vi "Parse Target ID.vi"(11 "targetID":string) -> (0 "target location":string, 3 "target name":string)   [LabVIEW 2020, in "NI_TargetHelper.lvlib"]
uses:
  <vilib>/TargetSupport/NI_TargetHelper/NI_TargetHelper.lvlib
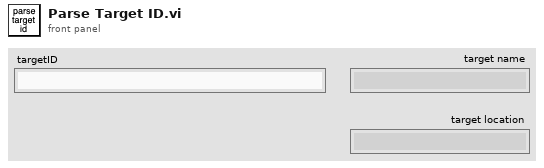
[diagram p1: front panel]
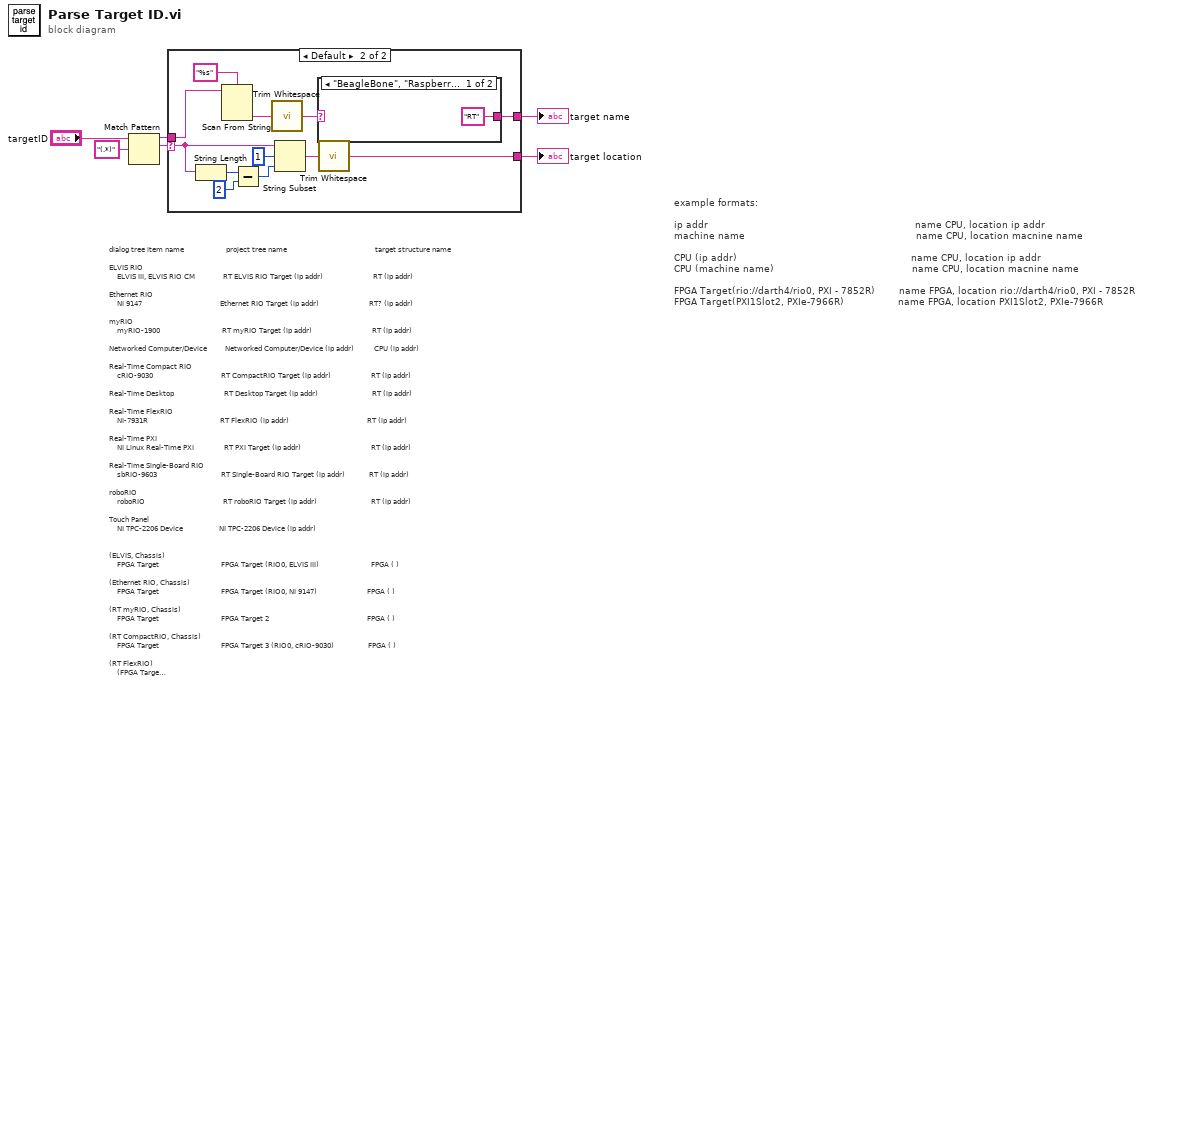
[diagram p0: block diagram]
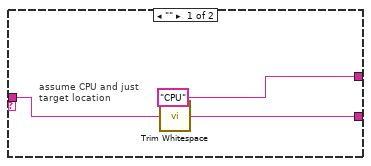
[diagram p2: hidden frame]
diagram:
  # "dialog tree item name                     project tree name                                            target structure name\n\nELVIS RIO\n    ELVIS III, ELVIS RIO CM              RT ELVIS RIO Target (ip addr)                         RT (ip addr)\n \nEthernet RIO\n    NI 9147                                       Ethernet RIO Target (ip addr)                         RT? (ip addr)\n\nmyRIO\n    myRIO-1900                               RT myRIO Target (ip addr)                              RT (ip addr)\n\nNetworked Computer/Device         Networked Computer/Device (ip addr)          CPU (ip addr)\n\nReal-Time Compact RIO\n    cRIO-9030                                  RT CompactRIO Target (ip addr)                    RT (ip addr)\n\nReal-Time Desktop                         RT Desktop Target (ip addr)                           RT (ip addr)\n\nReal-Time FlexRIO\n    NI-7931R                                    RT FlexRIO (ip addr)                                       RT (ip addr)\n\nReal-Time PXI\n    NI Linux Real-Time PXI               RT PXI Target (ip addr)                                   RT (ip addr)\n\nReal-Time Single-Board RIO\n    sbRIO-9603                                RT Single-Board RIO Target (ip addr)            RT (ip addr)\n\nroboRIO\n    roboRIO                                       RT roboRIO Target (ip addr)                           RT (ip addr)\n\nTouch Panel\n    NI TPC-2206 Device                  NI TPC-2206 Device (ip addr)\n\n\n(ELVIS, Chassis)\n    FPGA Target                               FPGA Target (RIO0, ELVIS III)                          FPGA ( )\n\n(Ethernet RIO, Chassis)\n    FPGA Target                               FPGA Target (RIO0, NI 9147)                         FPGA ( )\n\n(RT myRIO, Chassis)\n    FPGA Target                               FPGA Target 2                                                 FPGA ( )\n\n(RT CompactRIO, Chassis)\n    FPGA Target                               FPGA Target 3 (RIO0, cRIO-9030)                 FPGA ( )\n\n(RT FlexRIO)\n    (FPGA Target)                            FPGA Target 4 (RIO0, NI-7931R)                   FPGA ( )\n\n(RT PXI)\n    PXI-7951R                                 FPGA Target 5 (PXI-7951R)                           FPGA (slot no)\n\n(RT Single-Board RIO, Chassis)\n    FPGA Target                               FPGA Target 6 (RIO0, sbRIO-9603)               FPGA ( )\n\n(RT roboRIO, Chassis)\n    FPGA Target                               FPGA Target 7 (RIO0, roboRIO)                      FPGA ( )"
  # "example formats:\n\nip addr                                                                     name CPU, location ip addr\nmachine name                                                         name CPU, location macnine name\n\nCPU (ip addr)                                                          name CPU, location ip addr\nCPU (machine name)                                              name CPU, location macnine name\n\nFPGA Target(rio://darth4/rio0, PXI - 7852R)        name FPGA, location rio://darth4/rio0, PXI - 7852R\nFPGA Target(PXI1Slot2, PXIe-7966R)                  name FPGA, location PXI1Slot2, PXIe-7966R"
  n1 = Match Pattern(string="targetID", regular expression="(.*)") -> (before substring=w4:string, match substring=w5:string)  [unwired: 1 in, 2 out]
  n2 = case shown="Default" w5 {
    selector: w5 -> [_ w19]
    tunnel: w4 -> [w7 w12]
    tunnel: ["CPU" ("trimmed string") w10] -> w2
    tunnel: [w8 w15] -> w1
    frame "" {
      # "assume CPU and just\ntarget location"
      n3 = call <vilib>:"Trim Whitespace.vi"("string"=w7) -> ("trimmed string"=w8:string)  [unwired: 1 in]
    }
    frame Default {
      n4 = String Length(string=w19) -> (length=w20:i32)
      n5 = Scan From String(format string="%s", input string=w12) -> (output 1=w13:string)  [unwired: 3 in, 3 out]
      n6 = Subtract(x=w20, y=2) -> (x-y=w18:i32)
      n7 = call <vilib>:"Trim Whitespace.vi"("string"=w13) -> ("trimmed string"=w11:string)  [unwired: 1 in]
      n8 = String Subset(string=w19, offset (0)=1, length (rest)=w18) -> (substring=w16:string)
      n9 = case shown="\"BeagleBone\", \"Raspberry\"" w11 {
        selector: w11 -> [_ w23]
        tunnel: ["RT" w23] -> w10
        frame "BeagleBone", "Raspberry" {
        }
        frame Default {
        }
      }
      n10 = call <vilib>:"Trim Whitespace.vi"("string"=w16) -> ("trimmed string"=w15:string)  [unwired: 1 in]
    }
  }
  "target name" <- w2
  "target location" <- w1
